vi "Current_Time.vi"() -> (1 "Abs_Time.lvclass":refnum<class "Abs_Time.lvclass">)   [LabVIEW 2021]
uses:
  Abs_Types/Time/Abs_Time.lvclass
  Support/Curr_Time/Const_Current Time.lvclass
  C:/Users/Tim/Documents/GitHub/LV_Abstract/Source/Abs_Types/Time/Abs_Time.lvclass
  C:/Users/Tim/Documents/GitHub/LV_Abstract/Source/Abs_Types/Numeric/Abs_Numeric.lvclass
  C:/Users/Tim/Documents/GitHub/LV_Abstract/Source/Abs_Types/Value/Abs_Value.lvclass
  C:/Users/Tim/Documents/GitHub/LV_Abstract/Source/Abs_Types/Type/Abs_Type.lvclass
  C:/Users/Tim/Documents/GitHub/LV_Abstract/Source/Constants/Support/Curr_Time/Const_Current Time.lvclass
  C:/Users/Tim/Documents/GitHub/LV_Abstract/Source/Constants/Support/Interface/Const_Intf.lvclass
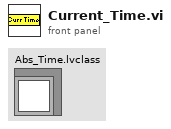
[diagram p1: front panel]
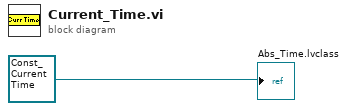
[diagram p0: block diagram]
diagram:
  "Abs_Time.lvclass" <- refnum<class "Const_Current Time.lvclass"> refnum ("Const_Current Time.lvclass")
